vi "TestBuilderFactory.vi"(8 "error in (no error)":errorcluster, 10 "Name":string) -> (0 "error out":errorcluster, 3 "Test Builder":refnum<class "TestBuilder.lvclass">)   [LabVIEW 2019]
doc: "Creates a TestBuilder object from the specified name."
uses:
  LVUnitTestBuilder/LVUnitTestBuilder.lvclass
  <vilib>/ErrorRing/Error Ring.xnode
  <vilib>/Utility/error.llb/Error Cluster From Error Code.vi
  C:/Users/de200256/Code/neuperger/lvunit/TestBuilder/TestBuilder.lvclass
  TestBuilder/TestBuilder.lvclass
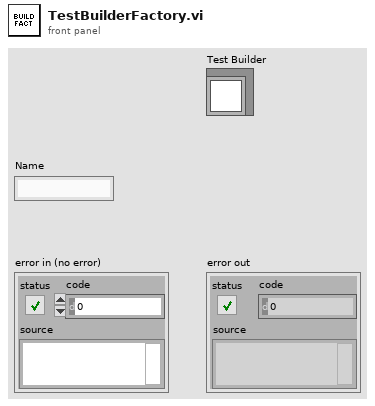
[diagram p1: front panel]
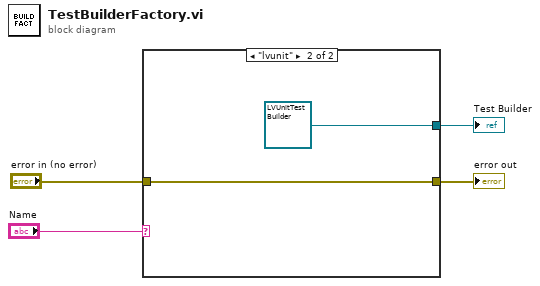
[diagram p0: block diagram]
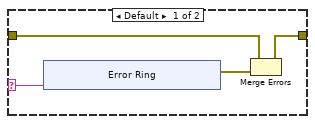
[diagram p2: hidden frame]
diagram:
  n1 = case shown="\"lvunit\"" "Name" {
    selector: "Name" -> [w8 _]
    tunnel: [w6 w17] -> w3
    tunnel: "error in (no error)" -> [w5 w17]
    tunnel: [_ refnum<class "LVUnitTestBuilder.lvclass"> refnum ("LVUnitTestBuilder")] -> w1
    frame Default {
      n2 = xnode "Error Ring"("parameter 0"=w8) -> ("error out"=w7:errorcluster)
      n3 = Merge Errors(w5, w7) -> (w6:errorcluster)
    }
    frame "lvunit" {
    }
  }
  "Test Builder" <- w1
  "error out" <- w3
